vi "RC_test_2.vi"() -> ()   [LabVIEW 2013]
uses:
  Data/TypeDefs/Rudder Set Suggestions.ctl
  Data/TypeDefs/DynamixelCycleTracker.ctl
  <vilib>/FPGAPlugInAG/myRIO-1900/niLvFpga_Open_myRIO-1900.vi
  <vilib>/rvi/interface/common/dynamic/niFpgaDynamicAddResources.vi
  <vilib>/rvi/interface/nirviOpenFPGA/nirviOpenFPGA.xnode
  FPGA Bitfiles/AutonomousSailbo_FPGATarget_myRIOPWMDecoder_0snwDOwOU4s.lvbitx
  FPGA_Code/myRIO_PWM_Decoder.vi
  <instrlib>/Dynamixel Motor/Dynamixel Motor.lvlib
panel:
  out "Write loop\ncounter":i32
  in  "Read actions per\nwrite action":i32=4
  out "Commanded sail value":dbl
  in  "VISA resource name":refnum<visa-resource-name>="ASRL3::INSTR"
  in  "Stop reading/writing":bool
  out "Read loop counter":i32
  out "Dynamixel\nPositions (deg)":dbl[](array[numeric])
  out "Updated Dynamixel Cycles":T1
  in  "Motors Enabled":bool[](array[boolean])=[TRUE, TRUE, TRUE]
  out "Commanded rudder value":T2 min=-0.95 max=0.95 scale=1.0..-1.0
  out "Motors IDs Found":u8[](array[numeric])
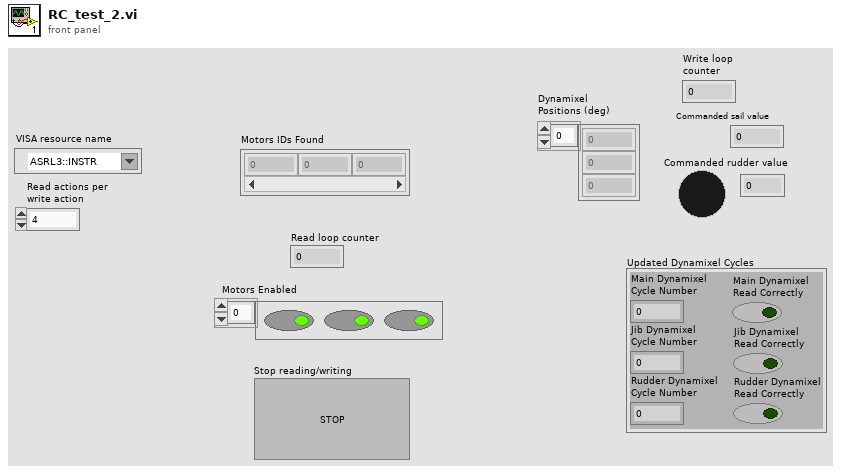
[diagram p1: front panel]
types:
  T1 = typedef "DynamixelCycleTracker.ctl" = cluster{"Main Dynamixel\nCycle Number":i32, "Jib Dynamixel\nCycle Number":i32, "Rudder Dynamixel\nCycle Number":i32, "Main Dynamixel\nRead Correctly":bool, "Jib Dynamixel\nRead Correctly":bool, "Rudder Dynamixel\nRead Correctly":bool}
  T2 = typedef "Rudder Set Suggestions.ctl" = dbl
  T3 = typedef "MotorSetup.ctl" = cluster{"Main Dynamixel Set Data":T4, "Rudder Dynamixel Set Data":T4, "Jib Dynamixel Set Data":T4}
  T4 = typedef "DynamixelSetupInfo.ctl" = cluster{"Lower Winch Bound (deg)":dbl, "Upper Winch Bound (deg)":dbl}
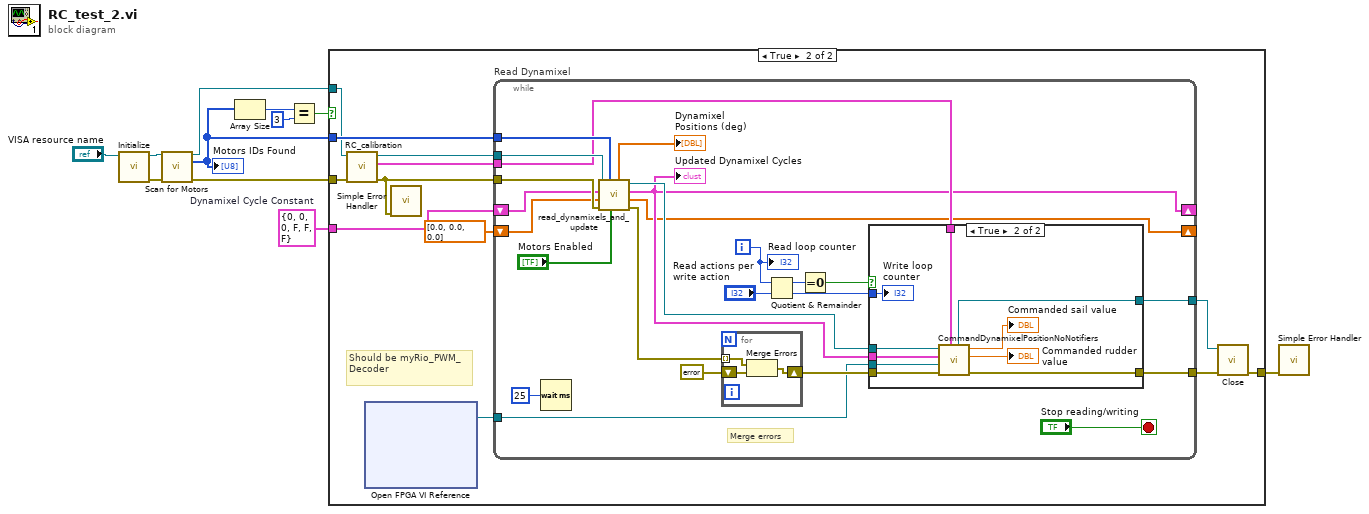
[diagram p0: block diagram]
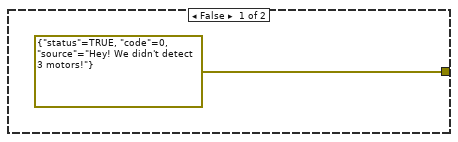
[diagram p2: hidden frame]
diagram:
  w4 = T1 {"Main Dynamixel\nCycle Number"=0, "Jib Dynamixel\nCycle Number"=0, "Rudder Dynamixel\nCycle Number"=0, "Main Dynamixel\nRead Correctly"=FALSE, "Jib Dynamixel\nRead Correctly"=FALSE, "Rudder Dynamixel\nRead Correctly"=FALSE}  # Dynamixel Cycle Constant
  n1 = call <instrlib>:"Initialize.vi"("VISA resource name"="VISA resource name") -> ("error out"=w2:errorcluster, "VISA resource name out"=w3:refnum<visa-resource-name>)  [unwired: 9 in]
  n2 = call <instrlib>:"Scan for Motors.vi"("VISA resource name"=w3, "error in (no error)"=w2) -> ("VISA resource name out"=w5:refnum<visa-resource-name>, "Motors IDs Found"=w11:u8[], "error out"=w6:errorcluster)  [unwired: 11 in]
  "Motors IDs Found" <- w11
  n3 = Array Size(array=w11) -> (size(s)=w7:i32)
  n4 = Equal?(x=w7, y=3) -> (x = y?=w8:bool)
  n5 = case shown="True" w8 {
    tunnel: w4 -> [_ w24]
    tunnel: w11 -> [_ w23]
    tunnel: w5 -> [_ w21]
    tunnel: w6 -> [_ w20]
    tunnel: [errorcluster {"status"=TRUE, "code"=0, "source"="Hey! We didn't detect 3 motors!"} ("error IO") w13] -> w10
    frame False {
    }
    frame True {
      # "Should be myRio_PWM_Decoder"
      n6 = call "RC_calibration.vi"("error in (no error)"=w20, "VISA resource name"=w21) -> ("error IO"=w18:errorcluster, "Dynamixel Bounds Out"=w15:T3, "VISA resource name out"=w19:refnum<visa-resource-name>)  [unwired: 7 in]
      n7 = xnode "Open FPGA VI Reference"() -> ("FPGA VI Reference Out"=w17:refnum<k20>)  [unwired: 2 in, 1 out]
      n8 = call <vilib>:"Simple Error Handler.vi"("error in (no error)"=w18) -> ()  [unwired: 4 in, 5 out]
      n9 = while "Read Dynamixel" {
        tunnel: w19 -> [w47]
        shift-right: [w28] -> _
        shift-left: w24 -> [w42]
        tunnel: w23 -> [w45]
        tunnel: w18 -> [w48]
        shift-right: [w26] -> _
        shift-left: dbl[] [0.0, 0.0, 0.0] -> [w43]
        tunnel: w17 -> [w39]
        tunnel: w15 -> [w38]
        tunnel: [w35] -> w14
        tunnel: [w34] -> w16
        i -> [w33]
        stop <- "Stop reading/writing" stop-if-true
        # "Merge errors"
        n10 = Wait (ms)(milliseconds to wait=u32 25) -> ()  [unwired: 1 out]
        n11 = call "read_dynamixels_and_update.vi"("Motors Enabled"="Motors Enabled", "Motors IDs Found"=w45, "error in (no error)"=w48, "Last read positions"=w43, "Dynamixel Cycle Constant"=w42, "VISA Refnum in"=w47) -> ("error out"=w25:errorcluster[], "Latest read positions (dyn)"=w26:dbl[], "Updated Dynamixle Cycles"=w28:T1, "VISA Refnum out"=w37:refnum<visa-resource-name>, "Dynamixel\nPositions (deg)"=→"Dynamixel\nPositions (deg)":dbl[])  [unwired: 1 in]
        "Updated Dynamixel Cycles" <- w28
        n12 = for {
          shift-right: [w63] -> w40
          shift-left: errorcluster {"status"=FALSE, "code"=0, "source"=""} ("error IO") -> [w62]
          tunnel: w25 -> [w61] mode=indexing
          n13 = Merge Errors(w61, w62) -> (w63:errorcluster)
        }
        n14 = Quotient & Remainder(x=w33, y="Read actions per\nwrite action") -> (x-y*floor(x/y)=w31:i32, floor(x/y)=w29:i32)
        n15 = Equal To 0?(x=w31) -> (x = 0?=w30:bool)
        n16 = case shown="True" w30 {
          tunnel: w40 -> [w50 w60]
          tunnel: w39 -> [_ w59]
          tunnel: w38 -> [_ w58]
          tunnel: w37 -> [w49 w57]
          tunnel: w28 -> [_ w56]
          tunnel: [w50 w53] -> w35
          tunnel: [w49 w52] -> w34
          tunnel: w29 -> [_ w51]
          frame False {
          }
          frame True {
            n17 = call "CommandDynamixelPositionNoNotifiers.vi"("Dynamixel Bounds"=w58, "error in"=w60, "FPGA VI Reference In"=w59, "Dynamixel Cycles"=w56, "VISA resource name"=w57) -> ("Error out"=w53:errorcluster, "Commanded rudder value"=→"Commanded rudder value":T2, "Debug sail value"=→"Commanded sail value":dbl, "VISA resource name OUT"=w52:refnum<visa-resource-name>)  [unwired: 3 in]
            "Write loop\ncounter" <- w51
          }
        }
        "Read loop counter" <- w33
      }
      n18 = call <instrlib>:"Close.vi"("error in (no error)"=w14, "VISA resource name"=w16) -> ("error out"=w13:errorcluster)  [unwired: 9 in]
    }
  }
  n19 = call <vilib>:"Simple Error Handler.vi"("error in (no error)"=w10) -> ()  [unwired: 4 in, 5 out]
